vi "FixMacPath.vi"(5 "Input Path String":string) -> (2 "Output Path":path)   [LabVIEW 2010]
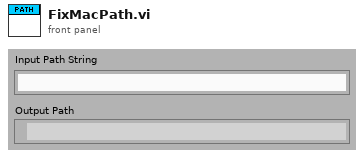
[diagram p1: front panel]
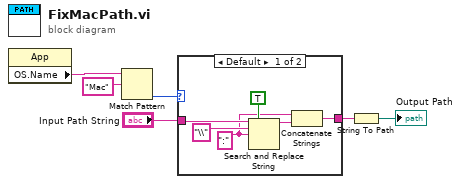
[diagram p0: block diagram]
diagram:
  n1 = property class="App"() -> ("OS.Name"=w6:string)  [unwired: 2 in, 2 out]
  n2 = Match Pattern(string=w6, regular expression="Mac") -> (offset past match=w4:i32)  [unwired: 1 in, 3 out]
  n3 = case shown="Default" w4 {
    tunnel: "Input Path String" -> [w12 w13]
    tunnel: [w7 w13] -> w2
    frame Default {
      w8 = ":" ("replace string (\"\")")
      n4 = Search and Replace String(replace all?=TRUE ("replace all? (F)"), input string=w12, search string="\\" ("replace string (\"\")"), replace string=w8) -> (result string=w9:string)  [unwired: 4 in, 3 out]
      n5 = Concatenate Strings(w8, w9) -> (w7:string)
    }
    frame -1 {
    }
  }
  n6 = String To Path(string=w2) -> (path=→"Output Path":path)
